vi "Angle Distance-old.vi"(1 "Target Angle":dbl(knob) scale=-180.0..180.0, 2 "Current Angle":dbl(knob) scale=-180.0..180.0) -> (0 "Distance":dbl)   [LabVIEW 2019]
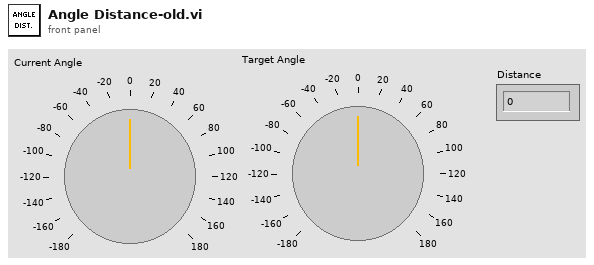
[diagram p1: front panel]
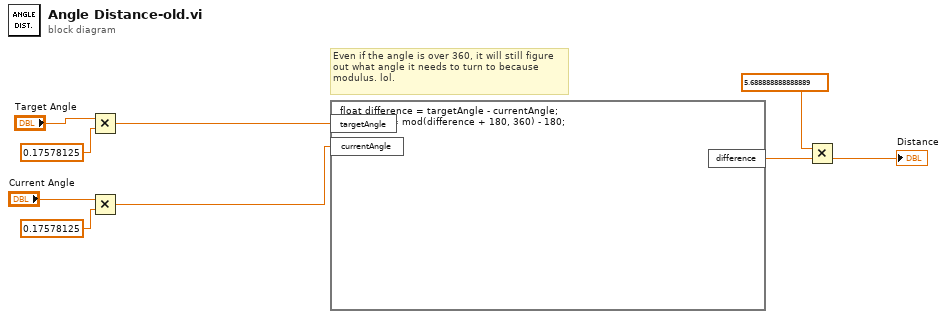
[diagram p0: block diagram]
diagram:
  # "Even if the angle is over 360, it will still figure\nout what angle it needs to turn to because \nmodulus. lol."
  n1 = Multiply(x="Target Angle", y=0.17578125) -> (x*y=w2:dbl)
  n2 = Multiply(x="Current Angle", y=0.17578125) -> (x*y=w7:dbl)
  n3 = formula code="float difference = targetAngle - currentAngle;\ndifference = mod(difference + 180, 360) - 180;"("targetAngle"=w2, "currentAngle"=w7) -> ("difference"=w8:dbl)
  n4 = Multiply(x=5.688888888888889, y=w8) -> (x*y=→"Distance":dbl)
